vi "Error Query.vi"(8 "error in (no error)":errorcluster, 11 "VISA resource name":refnum<visa-resource-name>) -> (0 "error out":errorcluster, 1 "Error Message":string, 2 "Error Code":i32, 3 "VISA resource name out":refnum<visa-resource-name>)   [LabVIEW 2017, in "Temptronic TP04300.lvlib"]
doc: "This VI reads a device-specific error code from the instrument's error queue."
uses:
  Temptronic TP04300.lvlib
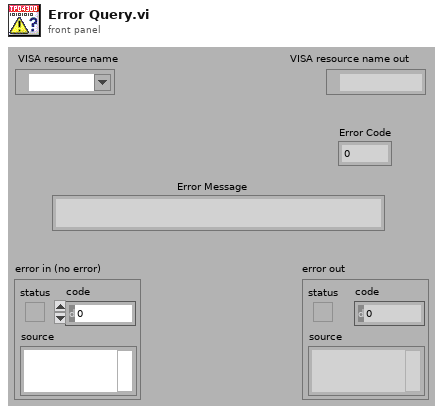
[diagram p1: front panel]
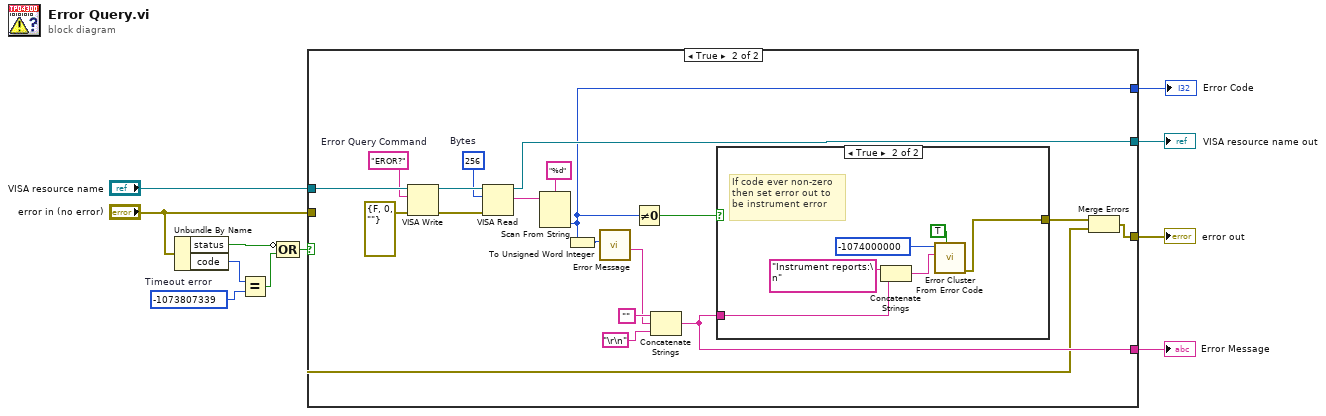
[diagram p0: block diagram]
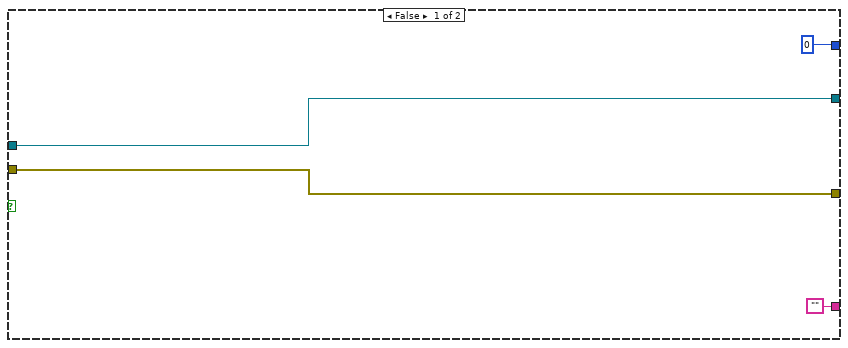
[diagram p2: hidden frame]
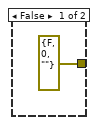
[diagram p3: hidden frame]
diagram:
  w6 = -1073807339  # Timeout error
  n1 = Unbundle By Name("error in (no error)") -> ("status"=w7:bool, "code"=w4:i32)
  n2 = Equal?(x=w4, y=w6) -> (x = y?=w5:bool)
  n3 = Compound Arithmetic op=OR(invert w7, w5) -> (w3:bool)
  n4 = case shown="True" w3 {
    tunnel: [w15 w34] -> w11
    tunnel: "VISA resource name" -> [w15 w33]
    tunnel: "error in (no error)" -> [w14 w27]
    tunnel: [w14 w31] -> w9
    tunnel: ["" w28] -> w2
    tunnel: [0 w16] -> w1
    frame False {
    }
    frame True {
      w25 = u32 256  # Bytes
      w23 = "EROR?"  # Error Query Command
      n5 = VISA Write(VISA resource name=w33, write buffer=w23, error in (no error)=errorcluster {"status"=FALSE, "code"=0, "source"=""}) -> (VISA resource name out=w26:refnum<visa-resource-name>, error out=w24:errorcluster)  [unwired: 1 out]
      n6 = VISA Read(VISA resource name=w26, byte count=w25, error in (no error)=w24) -> (VISA resource name out=w34:refnum<visa-resource-name>, read buffer=w21:string)  [unwired: 2 out]
      n7 = Scan From String(format string="%d", input string=w21) -> (output 1=w16:i32)  [unwired: 3 in, 3 out]
      n8 = To Unsigned Word Integer(number=w16) -> (unsigned 16bit integer=w19:u16)
      n9 = call "Error Message.vi"("Error Code in"=w19) -> ("Error Message"=w18:string)  [unwired: 8 in, 2 out]
      n10 = Not Equal To 0?(x=w16) -> (x != 0?=w17:bool)
      n11 = Concatenate Strings("", w18, "\r\n") -> (w28:string)
      n12 = case shown="True" w17 {
        tunnel: w28 -> [_ w40]
        tunnel: [errorcluster {"status"=FALSE, "code"=0, "source"=""} ("error out") w36] -> w30
        frame False {
        }
        frame True {
          # "If code ever non-zero\nthen set error out to\nbe instrument error"
          n13 = Concatenate Strings("Instrument reports:\n" ("Source"), w40) -> (w37:string)
          n14 = call <vilib>:"Error Cluster From Error Code.vi"("show call chain? (False)"=TRUE, "error message (\"\")"=w37, "error code (0)"=-1074000000 ("Code")) -> ("error out"=w36:errorcluster)  [unwired: 6 in]
        }
      }
      n15 = Merge Errors(w30, w27) -> (w31:errorcluster)
    }
  }
  "VISA resource name out" <- w11
  "error out" <- w9
  "Error Message" <- w2
  "Error Code" <- w1
